vi "basic-adam-test.vi"() -> ()   [LabVIEW 2024]
uses:
  controls/command-enum.ctl
  <vilib>/Instr/_visa.llb/VISA Configure Serial Port (Instr).vi
  controls/depreciated/analog-data-cluster.ctl
  controls/depreciated/thermocouple-data-cluster.ctl
  controls/digital-output-cluster.ctl
panel:
  out "acknowledge char":string
  out "Digital Outputs":T1
  in  "DO Control":T1
  out "Bytes at Serial Port":u32
  out "Analog Data Out":T2
  out "read return":u32
  out "Thermocouples":T3
  out "data csv":string
  out "status":string
  in  "Command":T4
  out "write return":u32
  out "error out":errorcluster
  out "read buffer":string
  out "command":string
  in  "Stop":bool
  in  "send-command":bool
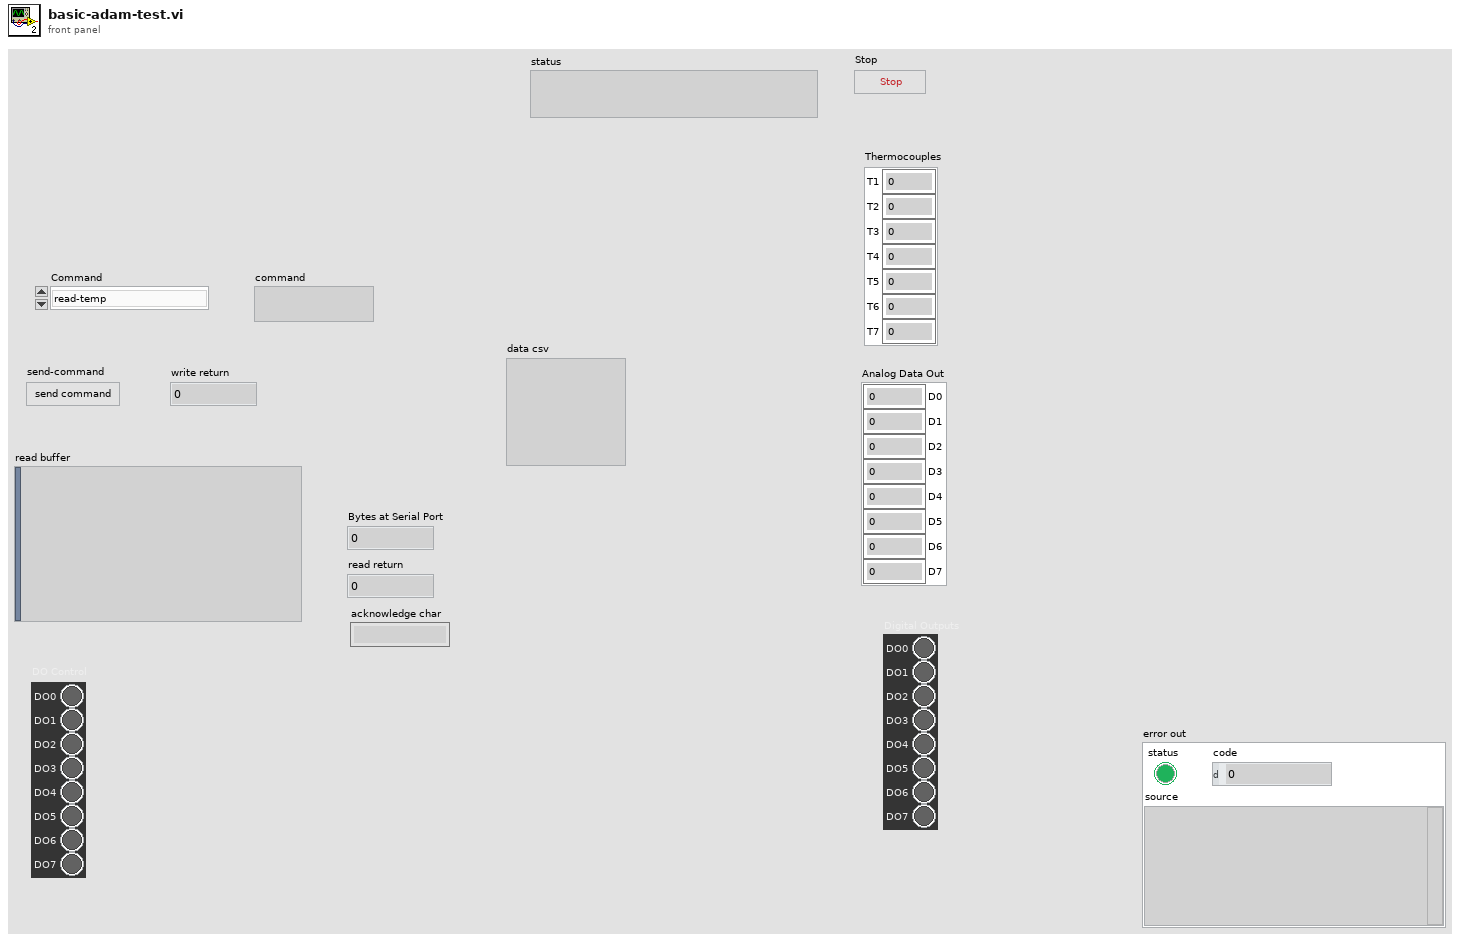
[diagram p1: front panel]
types:
  T1 = typedef "digital-output-cluster.ctl" = cluster{"DO0":bool, "DO1":bool, "DO2":bool, "DO3":bool, "DO4":bool, "DO5":bool, "DO6":bool, "DO7":bool}
  T2 = typedef "analog-data-cluster.ctl" = cluster{"D0":dbl, "D1":dbl, "D2":dbl, "D3":dbl, "D4":dbl, "D5":dbl, "D6":dbl, "D7":dbl}
  T3 = typedef "thermocouple-data-cluster.ctl" = cluster{"T1":dbl, "T2":dbl, "T3":dbl, "T4":dbl, "T5":dbl, "T6":dbl, "T7":dbl}
  T4 = typedef "command-enum.ctl" = enum16{"read-temp", "read-AI"}
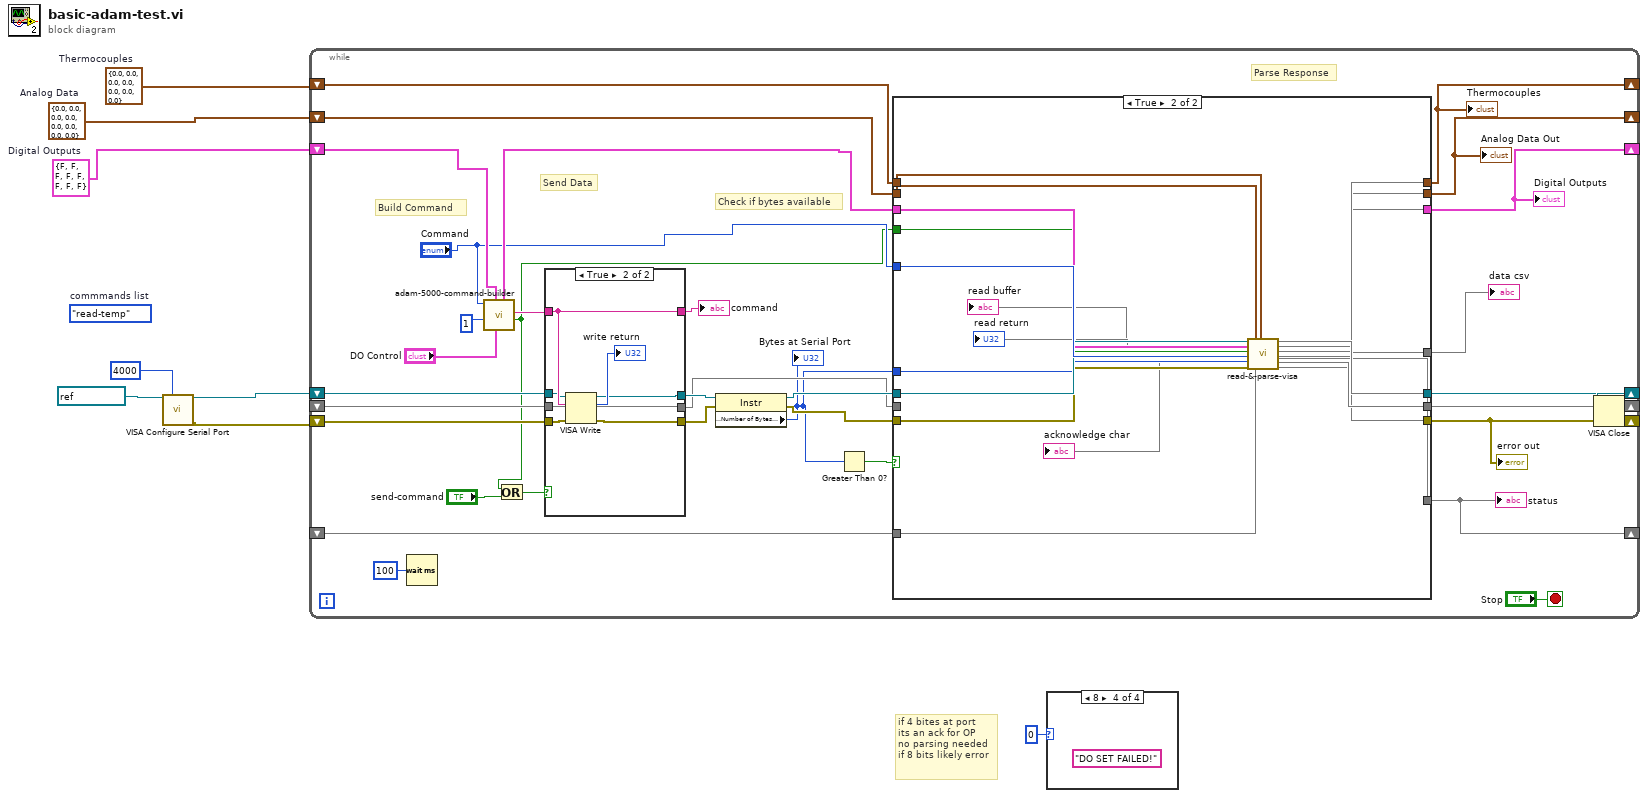
[diagram p0: block diagram]
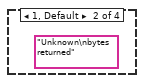
[diagram p3: hidden frame]
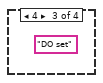
[diagram p4: hidden frame]
diagram:
  w2 = T1 {"DO0"=FALSE, "DO1"=FALSE, "DO2"=FALSE, "DO3"=FALSE, "DO4"=FALSE, "DO5"=FALSE, "DO6"=FALSE, "DO7"=FALSE}  # Digital Outputs
  w3 = T3 {"T1"=0.0, "T2"=0.0, "T3"=0.0, "T4"=0.0, "T5"=0.0, "T6"=0.0, "T7"=0.0}  # Thermocouples
  w4 = T2 {"D0"=0.0, "D1"=0.0, "D2"=0.0, "D3"=0.0, "D4"=0.0, "D5"=0.0, "D6"=0.0, "D7"=0.0}  # Analog Data
  (unwired) command-enum."read-temp"  # commmands list
  # "if 4 bites at port\nits an ack for OP\nno parsing needed\nif 8 bits likely error"
  n1 = call-poly "VISA Configure Serial Port"("VISA resource name"=refnum<visa-resource-name> "COM10", "timeout (10sec)"=u32 4000) -> ("VISA resource name out"=w9:refnum<visa-resource-name>, "error out"=w8:errorcluster)  [unwired: 12 in]
  n2 = while {
    shift-right: [w28] -> w6
    shift-left: w8 -> [w41]
    shift-right: [w36] -> w7
    shift-left: w9 -> [w42]
    shift-right: [w37] -> _
    shift-left: _ -> [w38]
    shift-right: [w31] -> _
    shift-left: w3 -> [w33]
    shift-right: [w34] -> _
    shift-left: _ -> [w32]
    shift-right: [w22] -> _
    shift-left: w4 -> [w29]
    shift-right: [w20] -> _
    shift-left: w2 -> [w18]
    stop <- "Stop" stop-if-true
    # "Check if bytes available"
    # "Parse Response"
    # "Send Data"
    # "Build Command"
    n3 = Wait (ms)(milliseconds to wait=u32 100) -> ()  [unwired: 1 out]
    n4 = call "adam-5000-command-builder.vi"("Output Control"="DO Control", "Current Output State"=w18, "ADAM-5000: Chassis ID"=u8 1, "Command"="Command") -> ("trigger write"=w11:bool, "Command Out"=w40:string, "DO Output"=w17:T1)  [unwired: 5 in]
    n5 = Or(x=w11, y="send-command") -> (x .or. y?=w19:bool)
    n6 = case shown="True" w19 {
      tunnel: w40 -> [w74 w80]
      tunnel: w41 -> [w71 w78]
      tunnel: [w74 w80] -> w39
      tunnel: w42 -> [w72 w79]
      tunnel: w38 -> [w73 w75]
      tunnel: [w72 w77] -> w27
      tunnel: [w71 w76] -> w26
      tunnel: [w73 w75] -> w24
      frame False {
      }
      frame True {
        n7 = VISA Write(VISA resource name=w79, write buffer=w80, error in (no error)=w78) -> (VISA resource name out=w77:refnum<visa-resource-name>, return count=→"write return":u32, error out=w76:errorcluster)
      }
    }
    "command" <- w39
    n8 = property class="Instr"(reference=w27, error in=w26) -> (reference out=w25:refnum<visa-resource-name>, error out=w23:errorcluster, "Serial Settings:Number of Bytes at Serial Port"=w14:u32)
    "Bytes at Serial Port" <- w14
    n9 = Greater Than 0?(x=w14) -> (x > 0?=w13:bool)
    n10 = case shown="True" w13 {
      tunnel: "Command" -> [_ w70]
      tunnel: w24 -> [w50 _]
      tunnel: [w50 w69] -> w37
      tunnel: w25 -> [w47 w59]
      tunnel: [w47 w68] -> w36
      tunnel: [w46 w67] -> w28
      tunnel: w23 -> [w46 w58]
      tunnel: [w50 w66] -> w35
      tunnel: [w49 w65] -> w31
      tunnel: [w44 w64] -> w34
      tunnel: w33 -> [w49 w62]
      tunnel: w32 -> [w44 w63]
      tunnel: w29 -> [w48 w61]
      tunnel: [w48 w60] -> w22
      tunnel: w14 -> [_ w57]
      tunnel: w17 -> [w45 w56]
      tunnel: [w45 w55] -> w20
      tunnel: w11 -> [_ w54]
      frame False {
      }
      frame True {
        n11 = call "read-&-parse-visa.vi"(0:w59, 1:w56, 2:w54, 3:w70, 4:w57, 5:w58, 6:w61, 7:w63, 8:w62) -> (9:→"acknowledge char", 10:→"read return", 11:w64, 12:→"read buffer", 13:w69, 14:w68, 15:w65, 16:w60, 17:w55, 18:w66, 19:w67)
      }
    }
    "status" <- w34
    "data csv" <- w35
    "Thermocouples" <- w31
    "Analog Data Out" <- w22
    "error out" <- w28
    "Digital Outputs" <- w20
  }
  n12 = case shown="8" u32 0 ("Bytes at Port") {
    frame 0 {
    }
    frame 1, Default {
      (unwired) "Unknown\nbytes returned" ("status")
    }
    frame 4 {
      (unwired) "DO set" ("status")
    }
    frame 8 {
      (unwired) "DO SET FAILED!" ("status")
    }
  }
  n13 = VISA Close(VISA resource name=w7, error in (no error)=w6) -> ()  [unwired: 1 out]
